vi "Read Until Char.vi"(8 "error in (no error)":errorcluster, 9 "Timeout(ms)":u16=500, 10 "Last Char":string="\r", 11 "VISA Refnum in":refnum<visa-resource-name>) -> (0 "error out":errorcluster, 1 "Delay":u32, 2 "String":string, 3 "VISA out":refnum<visa-resource-name>, 4 "Timed out":bool)   [LabVIEW 2018]
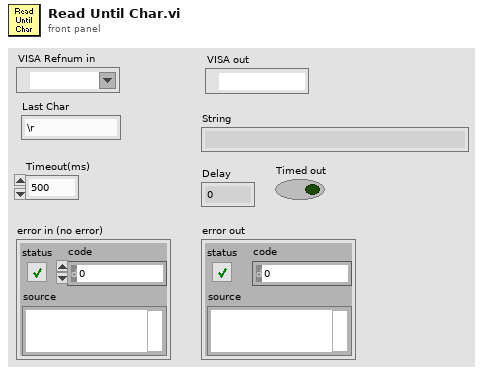
[diagram p1: front panel]
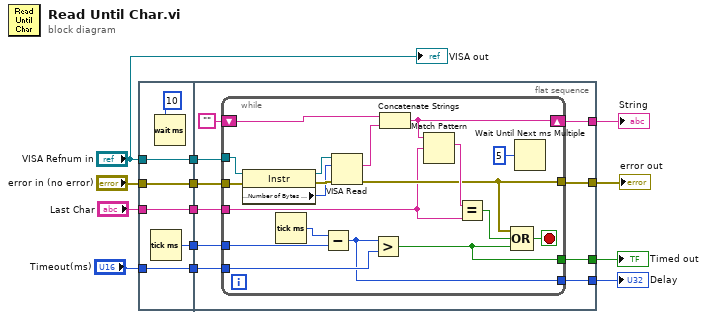
[diagram p0: block diagram]
diagram:
  n1 = flat-sequence {
    tunnel: "error in (no error)" -> [w17]
    tunnel: "Timeout(ms)" -> [w18]
    tunnel: "VISA Refnum in" -> [w19]
    tunnel: [w19] -> w13
    tunnel: [w18] -> w12
    tunnel: [w17] -> w11
    tunnel: [w16] -> w10
    tunnel: [w15] -> w3
    tunnel: "Last Char" -> [w15]
    tunnel: [w28] -> w4
    tunnel: [w27] -> w5
    tunnel: w13 -> [w29]
    tunnel: w12 -> [w26]
    tunnel: w11 -> [w25]
    tunnel: w10 -> [w23]
    tunnel: [w22] -> w8
    tunnel: [w21] -> w9
    tunnel: w3 -> [w20]
    frame #0 {
      n2 = Tick Count (ms)() -> (millisecond timer value=w16:u32)
      n3 = Wait (ms)(milliseconds to wait=u32 10) -> ()  [unwired: 1 out]
    }
    frame #1 {
      n4 = while {
        tunnel: [w39] -> w27
        tunnel: w26 -> [w34]
        tunnel: w25 -> [w44]
        tunnel: w29 -> [w47]
        shift-right: [w41] -> w28
        shift-left: "" -> [w43]
        tunnel: w23 -> [w35]
        tunnel: [w33] -> w22
        tunnel: [w32] -> w21
        tunnel: w20 -> [w31]
        stop <- w37 stop-if-true
        n5 = property class="Instr"(reference=w47, error in=w44) -> (reference out=w46:refnum<visa-resource-name>, error out=w48:errorcluster, "Serial Settings:Number of Bytes at Serial Port"=w45:u32)
        n6 = Tick Count (ms)() -> (millisecond timer value=w36:u32)
        n7 = Subtract(x=w36, y=w35) -> (x-y=w32:u32)
        n8 = VISA Read(VISA resource name=w46, byte count=w45, error in (no error)=w48) -> (read buffer=w42:string, error out=w39:errorcluster)  [unwired: 2 out]
        n9 = Greater?(x=w32, y=w34) -> (0:w33:bool)
        n10 = Concatenate Strings(w43, w42) -> (w41:string)
        n11 = Match Pattern(string=w41, regular expression=w31) -> (match substring=w40:string)  [unwired: 1 in, 3 out]
        n12 = Equal?(x=w40, y=w31) -> (x = y?=w38:bool)
        n13 = Compound Arithmetic op=OR(w39, w38, w33) -> (w37:bool)
        n14 = Wait Until Next ms Multiple(millisecond multiple=u32 5) -> ()  [unwired: 1 out]
      }
    }
  }
  "Delay" <- w9
  "Timed out" <- w8
  "error out" <- w5
  "String" <- w4
  "VISA out" <- "VISA Refnum in"
